vi "Load Multimeter Data.vi"(8 "error in":errorcluster, 11 "class objects":T1) -> (0 "error out":errorcluster, 3 "class objects":T1)   [LabVIEW 2011]
uses:
  Controls/Class Objects.ctl
  Modules/File/Configuration/Configuration.lvclass
  Modules/Hardware/Power Supply/Power Supply.lvclass
  Modules/Hardware/Mass Flow Controller/Mass Flow Controller.lvclass
  Modules/Hardware/PID/PID.lvclass
  Modules/Hardware/Valve Controller/Valve Controller.lvclass
  Modules/Hardware/Multimeter/Multimeter.lvclass
  Modules/Hardware/Vapour Generator/Vapour Generator.lvclass
  Modules/File/TDMS/TDMS.lvclass
  Modules/File/TDMS/Parameter Data Type.ctl
  Modules/File/TDMS/File Level.ctl
  Functional Global Data/Run Data.ctl
  Controls/TDMS File Handling.ctl
  Controls/User Interface Action.ctl
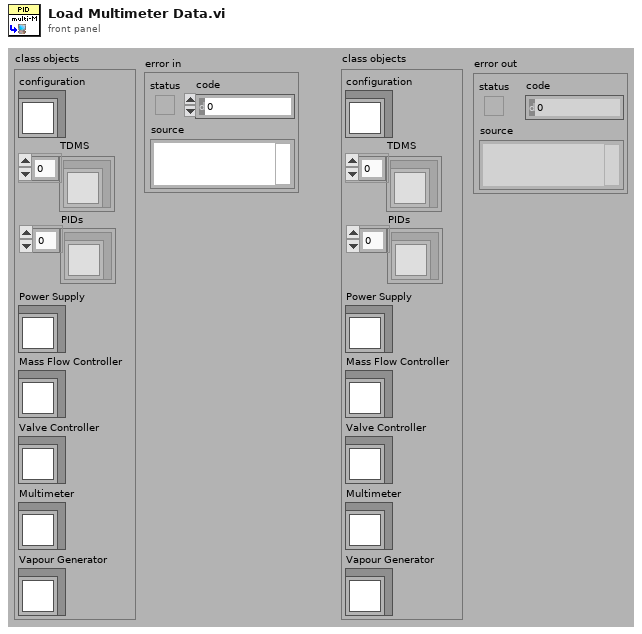
[diagram p1: front panel]
types:
  T1 = typedef "Class Objects.ctl" = cluster{"configuration":refnum<class "Configuration.lvclass">, "TDMS":refnum<class "TDMS.lvclass">[], "Power Supply":refnum<class "Power Supply.lvclass">, "Mass Flow Controller":refnum<class "Mass Flow Controller.lvclass">, "Valve Controller":refnum<class "Valve Controller.lvclass">, "Multimeter":refnum<class "Multimeter.lvclass">, "Vapour Generator":refnum<class "Vapour Generator.lvclass">, "PIDs":refnum<class "PID.lvclass">[]}
  T2 = typedef "TDMS.lvclass/Parameter Data Type.ctl" = enum16{"Boolean", "U32", "I32", "Double", "String", "Path"}
  T3 = typedef "TDMS.lvclass/File Level.ctl" = enum16{"File", "Group", "Channel"}
  T4 = typedef "Run Data.ctl" = enum16{"Initialize", "Add Sample Channel", "Set Run", "Get Number of Runs", "Set Run Params", "Get Spectrum", "Get Run Params", "Get Sample Params", "Get History", "Get Averaged History", "Get Run Param Names", "Set Run Param Names", "Get Sample Param Names", "Set Sample Param Names", "Get MFC Flow Rate Challenge Profile", "Get History Average"}
  T5 = typedef "TDMS File Handling.ctl" = enum16{"Add TDMS File", "Get Active TDMS File", "Set Active TDMS File", "Set Active TDMS File Index"}
  T6 = typedef "User Interface Action.ctl" = enum16{"Initialize", "Data Acquisition Disable", "Data View Disable", "Sample Set", "Sample Set 2D Data", "Sample Set x0 & dx", "Sample Add", "Sample Set Cursor", "Sample Set Offset & Multiplier", "Sample Set Axis Labels", "Sample Parameters Disabled", "Sample Parameters Update", "Run Update", "Run Set Offset & Multiplier", "Run Set Axis Labels", "Run Set Cursor", "Run Set Disabled", "Run Parameters Update", "Run Parameters Disabled", "Run Number Set", "Run Number Set Range", "Run Number Set Disabled", "Sample Number Set", "Sample Number Set Range", "Notes Set Value", "Update Plot", "Set Plot Parameters", "Update Concentration Plot", "Time Set", "Clear DAQ Display", "Clear Analysis Display", "Status Bar Set", "Progress Bar Set", "Display Mode Set", "Experiment Type Set", "Analysis Plot Average Set", "Stop"}
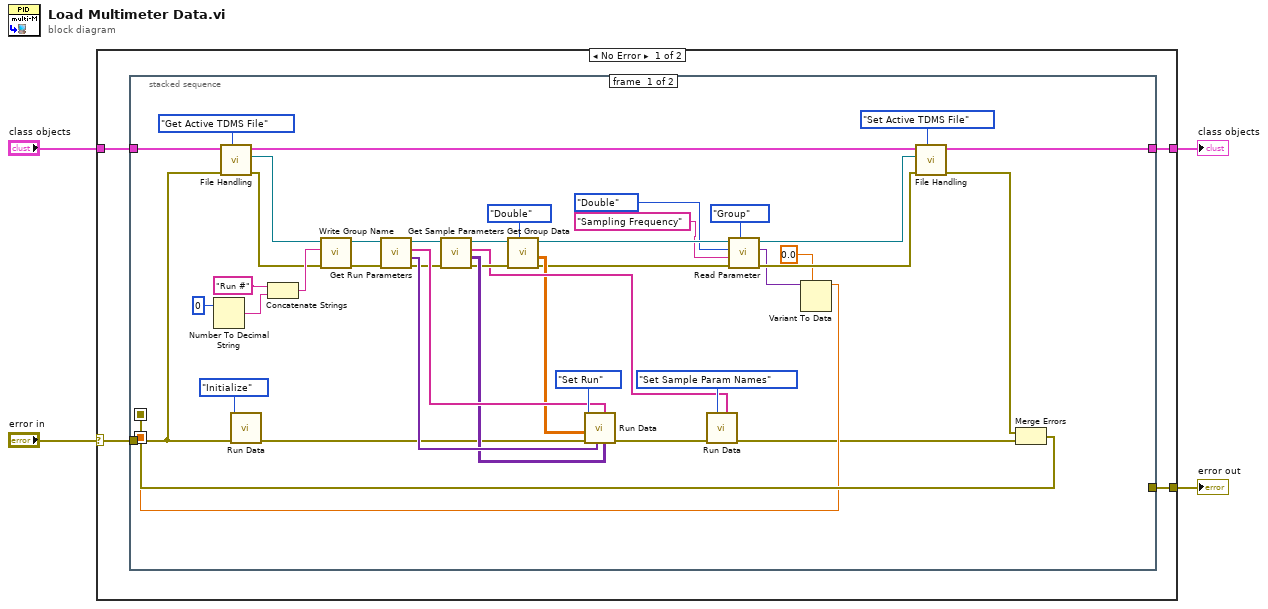
[diagram p0: block diagram]
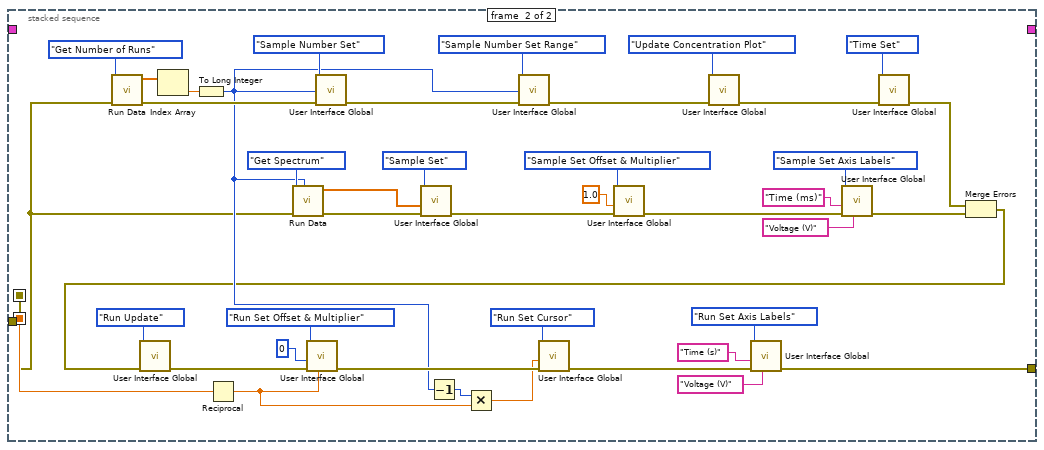
[diagram p2: hidden frame]
diagram:
  n1 = case shown="No Error" "error in" {
    selector: "error in" -> [w6 w93]
    tunnel: "class objects" -> [w8 w94]
    tunnel: [w5 w93] -> w3
    tunnel: [w7 w94] -> w2
    frame No Error {
      n2 = stacked-sequence {
        seq-local: [w21 _] -> [_ w54]
        seq-local: [w11 _] -> [_ w78]
        tunnel: w8 -> [w48 _]
        tunnel: [w44 _] -> w7
        tunnel: w6 -> [w40 _]
        tunnel: [_ w57] -> w5
        frame #0 {
          n3 = Number To Decimal String(number=0) -> (decimal integer string=w31:string)  [unwired: 1 in]
          n4 = call "File Handling.vi"("TDMS File Handling"=TDMS_File_Handling."Get Active TDMS File", "error in"=w40, "Class objects"=w48) -> ("error out"=w29:errorcluster, "TDMS File"=w47:refnum<class "TDMS.lvclass">, "Class objects"=w46:T1)  [unwired: 6 in]
          n5 = call "Run Data.vi"("error in"=w40, "action"=Run_Data."Initialize" ("Action")) -> ("error out"=w24:errorcluster)  [unwired: 6 in, 3 out]
          n6 = Concatenate Strings("Run #" ("string"), w31) -> (w30:string)
          n7 = call-dynamic "Write Group Name.vi"("error in (no error)"=w29, "Group Name"=w30, "TDMS in"=w47) -> ("error out"=w25:errorcluster, "TDMS out"=w23:refnum<class "TDMS.lvclass">)  [unwired: 7 in]
          n8 = call-dynamic "Get Run Parameters.vi"("error in"=w25, "TDMS in"=w23) -> ("error out"=w37:errorcluster, "run params"=w39:variant[], "param names"=w38:string[], "TDMS out"=w36:refnum<class "TDMS.lvclass">)  [unwired: 6 in]
          n9 = call-dynamic "Get Sample Parameters.vi"("error in"=w37, "TDMS in"=w36) -> ("error out"=w33:errorcluster, "sample params"=w34:variant[][], "sample param names"=w26:string[], "TDMS out"=w35:refnum<class "TDMS.lvclass">)  [unwired: 6 in]
          n10 = call "Get Group Data.vi"("data type"=enum16{"I16", "Double"}."Double" ("Data Type"), "error in"=w33, "TDMS in"=w35) -> ("error out"=w18:errorcluster, "double group data"=w22:dbl[][], "TDMS out"=w20:refnum<class "TDMS.lvclass">)  [unwired: 3 in, 3 out]
          n11 = call "Run Data.vi"("Params 2D IN"=w34, "Param Names IN"=w38, "Params 1D IN"=w39, "error in"=w24, "Data 2D IN"=w22, "action"=Run_Data."Set Run" ("Action")) -> ("error out"=w27:errorcluster)  [unwired: 2 in, 3 out]
          n12 = call "Run Data.vi"("Param Names IN"=w26, "error in"=w27, "action"=Run_Data."Set Sample Param Names") -> ("error out"=w10:errorcluster)  [unwired: 5 in, 3 out]
          n13 = call-dynamic "Read Parameter.vi"("file level"=File_Level."Group", "error in"=w18, "Parameter Name"="Sampling Frequency", "data type"=Parameter_Data_Type."Double", "TDMS in"=w20) -> ("error out"=w15:errorcluster, "parameter"=w13:variant, "TDMS out"=w14:refnum<class "TDMS.lvclass">)  [unwired: 3 in, 1 out]
          n14 = Variant To Data(type=0.0, Variant=w13) -> (data=w11:dbl)  [unwired: 1 in, 1 out]
          n15 = call "File Handling.vi"("TDMS File Handling"=TDMS_File_Handling."Set Active TDMS File", "error in"=w15, "TDMS File"=w14, "Class objects"=w46) -> ("error out"=w45:errorcluster, "Class objects"=w44:T1)  [unwired: 5 in, 1 out]
          n16 = Merge Errors(w45, w10) -> (w21:errorcluster)
        }
        frame #1 {
          n17 = call "Run Data.vi"("error in"=w54, "action"=Run_Data."Get Number of Runs" ("Action")) -> ("error out"=w63:errorcluster, "Data 1D OUT"=w62:dbl[])  [unwired: 6 in, 2 out]
          n18 = Index Array(array=w62) -> (element=w61:dbl)  [unwired: 1 in]
          n19 = To Long Integer(number=w61) -> (32bit integer=w59:i32)
          n20 = Reciprocal(x=w78) -> (1/x=w76:dbl)
          n21 = call "Run Data.vi"("Index Number"=w59, "error in"=w54, "action"=Run_Data."Get Spectrum" ("Action")) -> ("error out"=w92:errorcluster, "Data 1D OUT"=w89:dbl[])  [unwired: 5 in, 2 out]
          n22 = call "User Interface Global.vi"("error in"=w63, "data1"=w59, "action"=User_Interface_Action."Sample Number Set" ("Action")) -> ("error out"=w80:errorcluster)  [unwired: 8 in]
          n23 = call "User Interface Global.vi"("error in"=w92, "data1"=w89, "action"=User_Interface_Action."Sample Set" ("Action")) -> ("error out"=w87:errorcluster)  [unwired: 8 in]
          n24 = Decrement(x=w59) -> (x-1=w74:i32)
          n25 = Multiply(x=w74, y=w76) -> (x*y=w75:dbl)
          n26 = call "User Interface Global.vi"("error in"=w80, "data1"=w59, "action"=User_Interface_Action."Sample Number Set Range" ("Action")) -> ("error out"=w52:errorcluster)  [unwired: 8 in]
          n27 = call "User Interface Global.vi"("error in"=w87, "data1"=1.0, "action"=User_Interface_Action."Sample Set Offset & Multiplier" ("Action")) -> ("error out"=w67:errorcluster)  [unwired: 8 in]
          n28 = call "User Interface Global.vi"("error in"=w52, "action"=User_Interface_Action."Update Concentration Plot" ("Action")) -> ("error out"=w53:errorcluster)  [unwired: 9 in]
          n29 = call "User Interface Global.vi"("data2"="Voltage (V)", "error in"=w67, "data1"="Time (ms)", "action"=User_Interface_Action."Sample Set Axis Labels" ("Action")) -> ("error out"=w60:errorcluster)  [unwired: 7 in]
          n30 = call "User Interface Global.vi"("error in"=w53, "action"=User_Interface_Action."Time Set") -> ("error out"=w51:errorcluster)  [unwired: 9 in]
          n31 = Merge Errors(w51, w60) -> (w58:errorcluster)
          n32 = call "User Interface Global.vi"("error in"=w58, "action"=User_Interface_Action."Run Update" ("Action")) -> ("error out"=w79:errorcluster)  [unwired: 9 in]
          n33 = call "User Interface Global.vi"("data2"=w76, "error in"=w79, "data1"=0, "action"=User_Interface_Action."Run Set Offset & Multiplier" ("Action")) -> ("error out"=w81:errorcluster)  [unwired: 7 in]
          n34 = call "User Interface Global.vi"("error in"=w81, "data1"=w75, "action"=User_Interface_Action."Run Set Cursor" ("Action")) -> ("error out"=w72:errorcluster)  [unwired: 8 in]
          n35 = call "User Interface Global.vi"("data2"="Voltage (V)", "error in"=w72, "data1"="Time (s)", "action"=User_Interface_Action."Run Set Axis Labels" ("Action")) -> ("error out"=w57:errorcluster)  [unwired: 7 in]
        }
      }
    }
    frame Error {
    }
  }
  "class objects" <- w2
  "error out" <- w3
